vi "7.4-6.7.4-How Client.vi"() -> ()   [LabVIEW 2010]
doc: "This VI implements a client for the Named Service UDP Server.vi.\nIt connects to a service by specifying the server address and the name of the service. After sending a 'Hello' string to the server, the client receives the string sent by the server, displays the string and closes the connection.\n\n<b>Note:</b> This VI is built to work with the Named Service UDP Server.vi in UDP.llb."
uses:
  7.0-Global.vi
  6-OCU Neurons/6.4-How Reporting Typedef.ctl
  6-OCU Neurons/6.0-Super Heart Beat.ctl
panel:
  out "data":T1
  out "Super Heart Beat 2":T2
  out "Error":errorcluster
  in  "stop":bool
  out "Super Heart Beat":T2
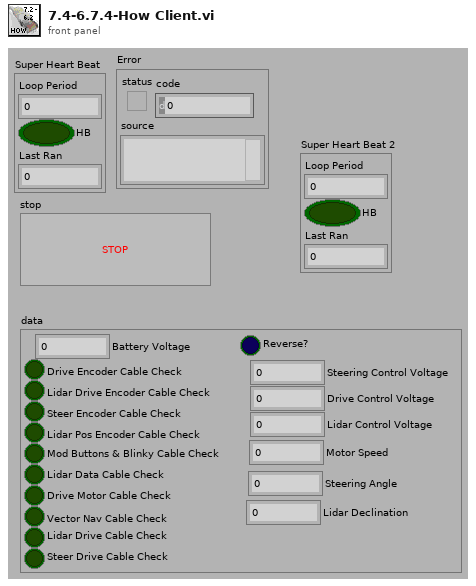
[diagram p1: front panel]
types:
  T1 = typedef "6.4-How Reporting Typedef.ctl" = cluster{"Motor Speed":i32, "Lidar Declination":i32, "Steering Angle":i32, "Battery Voltage":dbl, "Drive Encoder Cable Check":bool, "Lidar Drive Encoder Cable Check":bool, "Steer Encoder Cable Check":bool, "Lidar Pos Encoder Cable Check":bool, "Mod Buttons & Blinky Cable Check":bool, "Lidar Data Cable Check":bool, "Drive Motor Cable Check":bool, "Vector Nav Cable Check":bool, "Lidar Drive Cable Check":bool, "Steer Drive Cable Check":bool, "Reverse?":bool, "Steering Control Voltage":dbl, "Drive Control Voltage":dbl, "Lidar Control Voltage":dbl}
  T2 = typedef "6.0-Super Heart Beat.ctl" = cluster{"Loop Period":u32, "HB":bool, "Last Ran":u32}
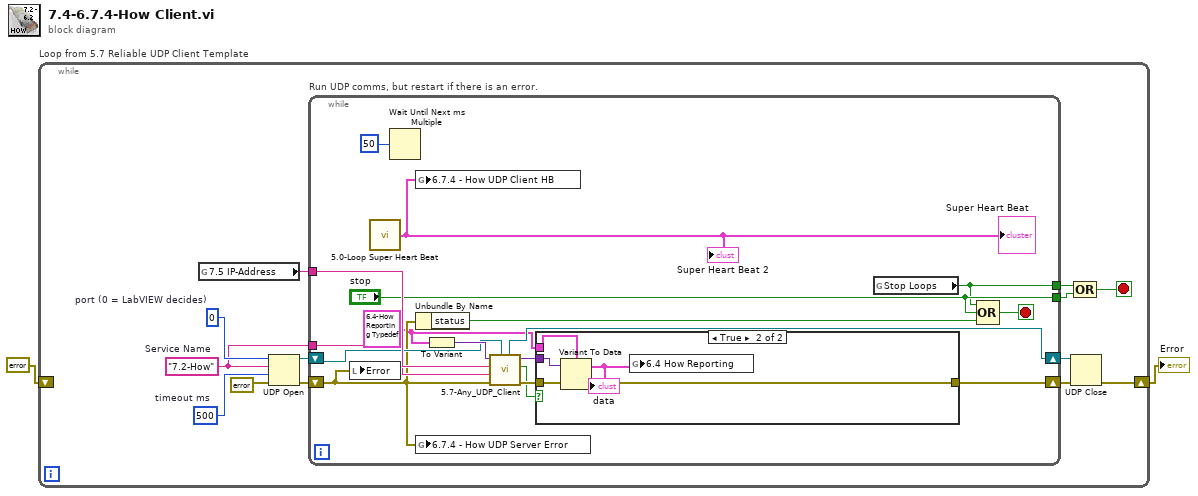
[diagram p0: block diagram]
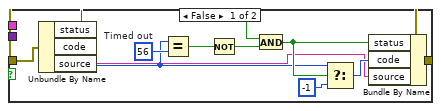
[diagram p2: hidden frame]
diagram:
  n1 = while "Loop from 5.7 Reliable UDP Client Template" {
    shift-right: [w8] -> w2
    shift-left: errorcluster {"status"=FALSE, "code"=0, "source"=""} ("error out") -> [_]
    stop <- w13 stop-if-true
    w5 = 500  # timeout ms
    w7 = u16 0  # port (0 = LabVIEW decides)
    w6 = "7.2-How"  # Service Name
    n2 = global read "7.0-Global.vi" "7.5 IP-Address"() -> (w3:string)
    n3 = UDP Open(8:errorcluster {"status"=FALSE, "code"=0, "source"=""} ("error in (no error)"), 9:w5, 10:w6, 11:w7) -> (port=w12:refnum<k16>, 0:w10:errorcluster)  [unwired: 1 in, 1 out]
    n4 = while "Run UDP comms, but restart if there is an error." {
      tunnel: w6 -> [w29]
      tunnel: w3 -> [w30]
      tunnel: [w19] -> w15
      tunnel: ["stop"] -> w14
      shift-right: [w23] -> w11
      shift-left: w12 -> [w24]
      shift-right: [w22] -> w9
      shift-left: w10 -> [w18]
      stop <- w32 stop-if-true
      w16 = T1 {"Motor Speed"=0, "Lidar Declination"=0, "Steering Angle"=0, "Battery Voltage"=0.0, "Drive Encoder Cable Check"=FALSE, "Lidar Drive Encoder Cable Check"=FALSE, "Steer Encoder Cable Check"=FALSE, "Lidar Pos Encoder Cable Check"=FALSE, "Mod Buttons & Blinky Cable Check"=FALSE, "Lidar Data Cable Check"=FALSE, "Drive Motor Cable Check"=FALSE, "Vector Nav Cable Check"=FALSE, "Lidar Drive Cable Check"=FALSE, "Steer Drive Cable Check"=FALSE, "Reverse?"=FALSE, "Steering Control Voltage"=0.0, "Drive Control Voltage"=0.0, "Lidar Control Voltage"=0.0} ("6.4 How Reporting")
      n5 = local write "Error"(w18) -> ()
      n6 = call "5.0-Loop Super Heart Beat.vi"() -> ("Super Heart Beat"=w17:T2)
      "Super Heart Beat" <- w17
      "Super Heart Beat 2" <- w17
      n7 = Wait Until Next ms Multiple(millisecond multiple=u32 50) -> ()  [unwired: 1 out]
      n8 = global write "7.0-Global.vi" "6.7.4 - How UDP Client HB"(w17) -> ()
      n9 = Unbundle By Name(w18) -> ("status"=w25:bool)
      n10 = global write "7.0-Global.vi" "6.7.4 - How UDP Server Error"(w18) -> ()
      n11 = To Variant(anything=w16) -> (Variant=w28:variant)
      n12 = call "5.7-Any_UDP_Client.vi"("Port In"=w24, "error In"=w18, "Max Size"=w29, 10:w30, "DataTypeIn"=w28) -> ("Error Out"=w21:errorcluster, "Check Passed"=w20:bool, "DataOut"=w27:variant, "Port out"=w23:refnum<k16>)  [unwired: 3 in]
      n13 = case "Ignore Timeouts" shown="True" w20 {
        tunnel: w27 -> [_ w48]
        tunnel: w16 -> [_ w45]
        tunnel: w21 -> [w43 w47]
        tunnel: [w42 w46] -> w22
        frame False {
          w41 = 56  # Timed out
          n14 = Unbundle By Name(w43) -> ("status"=w38:bool, "code"=w36:i32, "source"=w33:string)
          n15 = Equal?(x=w36, y=w41) -> (x = y?=w40:bool)
          n16 = Not(x=w40) -> (.not. x?=w39:bool)
          n17 = And(x=w38, y=w39) -> (x .and. y?=w37:bool)
          n18 = Select(t=w36, s=w37, f=-1) -> (s? t:f=w34:i32)
          n19 = Bundle By Name(cluster=w43, "status"=w37, "code"=w34, "source"=w33) -> (w42:errorcluster)
        }
        frame True {
          n20 = Variant To Data(error in=w47, Variant=w48, type=w45) -> (error out=w46:errorcluster, data=w44:T1)
          "data" <- w44
          n21 = global write "7.0-Global.vi" "6.4 How Reporting"(w44) -> ()
        }
      }
      n22 = global read "7.0-Global.vi" "Stop Loops"() -> (w19:bool)
      n23 = Compound Arithmetic op=OR(w19, "stop", w25) -> (w32:bool)
    }
    n24 = UDP Close(connection ID=w11, 8:w9) -> (error out=w8:errorcluster)  [unwired: 1 out]
    n25 = Compound Arithmetic op=OR(w15, w14) -> (w13:bool)
  }
  "Error" <- w2
